vi "Get Anchor Coordinates.vi"(8 "error in (no error)":errorcluster, 10 "Raw Coords":cluster{"X":i32, "Y":i32}, 11 "Bus in":refnum<class "Bus.lvclass">) -> (0 "error out":errorcluster, 2 "Anchor Coords":cluster{dbl, dbl}, 3 "Bus out":refnum<class "Bus.lvclass">)   [LabVIEW 2015, in "Bus.lvclass"]
uses:
  Bus.lvclass
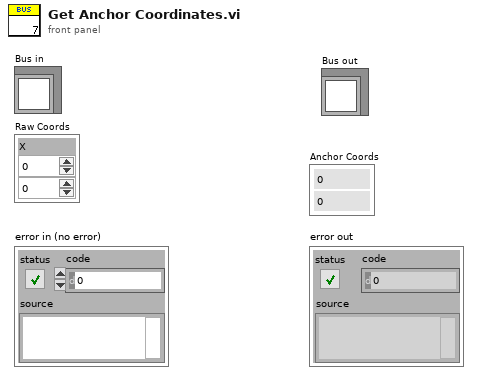
[diagram p1: front panel]
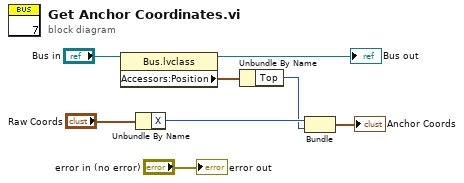
[diagram p0: block diagram]
diagram:
  n1 = property class="Bus.lvclass"(reference="Bus in") -> (reference out=→"Bus out":refnum<class "Bus.lvclass">, "Accessors:Position"=w7:cluster{"Left":i32, "Top":i32})  [unwired: 1 in, 1 out]
  n2 = Unbundle By Name("Raw Coords") -> ("X"=w5:i32)
  n3 = Unbundle By Name(w7) -> ("Top"=w4:i32)
  n4 = Bundle("X"=w5, "Top"=w4) -> (→"Anchor Coords":cluster{"X":i32, "Top":i32})  [unwired: 1 in]
  "error out" <- "error in (no error)"
